vi "MM6.ProcEvents.vi"(0 "i ref in":refnum<vi>, 5 "error in (no error)":errorcluster) -> (14 "i ref out":refnum<vi>, 19 "error out":errorcluster)   [LabVIEW 2014, in "MM6.lvlib"]
doc: "This method is used to define the events the object will listen to. Add your own events here."
uses:
  MM6.lvlib
  CS_Core/BaseProcess/BaseProcess.event definition.ctl
  CS_Core/CAEObj/CAEObj.event definition.ctl
  CS_Core/BaseProcess/BaseProcess.descriptor string definition.ctl
  CS_Core/BaseProcess/BaseProcess.lvlib
  CS_Core/CAEObj/CAEObj.lvlib
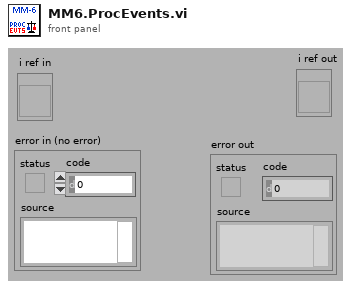
[diagram p1: front panel]
types:
  T1 = typedef "BaseProcess.lvlib/BaseProcess.event definition.ctl" = cluster{"CAEEvtDef":T2, "Data Descriptor":T3}
  T2 = typedef "CAEObj.lvlib/CAEObj.event definition.ctl" = cluster{"URL":string, "enable":bool, "ignoreResID":bool}
  T3 = typedef "BaseProcess.lvlib/BaseProcess.descriptor string definition.ctl" = string
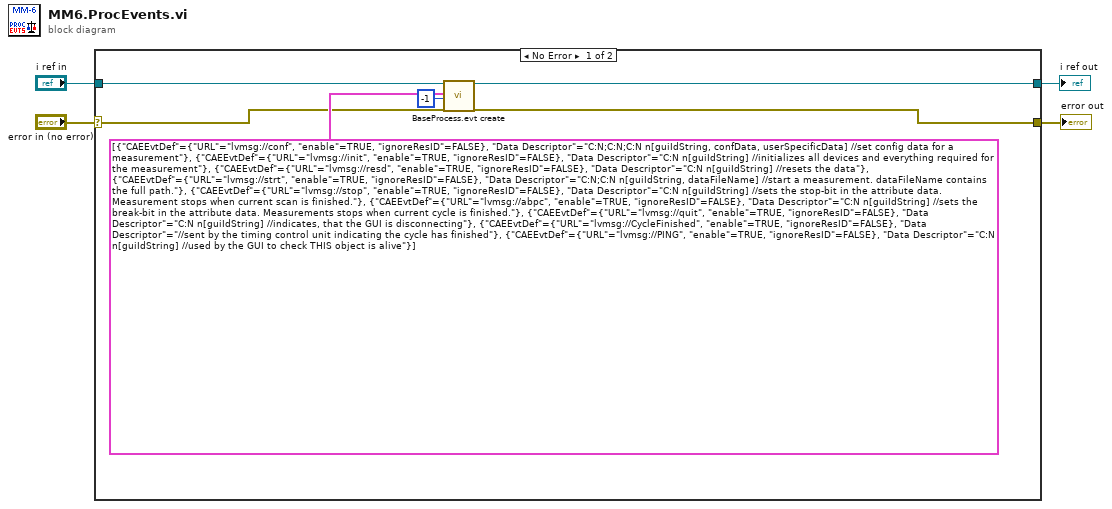
[diagram p0: block diagram]
diagram:
  n1 = case shown="No Error" "error in (no error)" {
    selector: "error in (no error)" -> [w6 w11]
    tunnel: "i ref in" -> [w10 w12]
    tunnel: [w8 w12] -> w3
    tunnel: [w7 w11] -> w2
    frame No Error {
      n2 = call "BaseProcess.evt create.vi"("i ref in"=w10, "newEvents"=T1[] [{"CAEEvtDef"={"URL"="lvmsg://conf", "enable"=TRUE, "ignoreResID"=FALSE}, "Data Descriptor"="C:N;C:N;C:N n[guiIdString, confData, userSpecificData] //set config data for a measurement"}, {"CAEEvtDef"={"URL"="lvmsg://init", "enable"=TRUE, "ignoreResID"=FALSE}, "Data Descriptor"="C:N n[guiIdString] //initializes all devices and everything required for the measurement"}, {"CAEEvtDef"={"URL"="lvmsg://resd", "enable"=TRUE, "ignoreResID"=FALSE}, "Data Descriptor"="C:N n[guiIdString] //resets the data"}, {"CAEEvtDef"={"URL"="lvmsg://strt", "enable"=TRUE, "ignoreResID"=FALSE}, "Data Descriptor"="C:N;C:N n[guiIdString, dataFileName] //start a measurement. dataFileName contains the full path."}, {"CAEEvtDef"={"URL"="lvmsg://stop", "enable"=TRUE, "ignoreResID"=FALSE}, "Data Descriptor"="C:N n[guiIdString] //sets the stop-bit in the attribute data. Measurement stops when current scan is finished."}, {"CAEEvtDef"={"URL"="lvmsg://abpc", "enable"=TRUE, "ignoreResID"=FALSE}, "Data Descriptor"="C:N n[guiIdString] //sets the break-bit in the attribute data. Measurements stops when current cycle is finished."}, {"CAEEvtDef"={"URL"="lvmsg://quit", "enable"=TRUE, "ignoreResID"=FALSE}, "Data Descriptor"="C:N n[guiIdString] //indicates, that the GUI is disconnecting"}, {"CAEEvtDef"={"URL"="lvmsg://CycleFinished", "enable"=TRUE, "ignoreResID"=FALSE}, "Data Descriptor"="//sent by the timing control unit indicating the cycle has finished"}, {"CAEEvtDef"={"URL"="lvmsg://PING", "enable"=TRUE, "ignoreResID"=FALSE}, "Data Descriptor"="C:N n[guiIdString] //used by the GUI to check THIS object is alive"}] ("new events"), "ms timeout (10000)"=-1, "error in (no error)"=w6) -> ("i ref out"=w8:refnum<vi>, "error out"=w7:errorcluster)  [unwired: 12 in, 2 out]
    }
    frame Error {
    }
  }
  "i ref out" <- w3
  "error out" <- w2
